vi "ex_readRawDataTDM.vi"(1 "read info in":T2, 5 "single values":bool, 7 "specified size":bool, 9 "segment size":i32, 11 "error in (no error)":errorcluster) -> (2 "read info out":T2, 6 "signals":waveform(dbl)[](array[waveform]), 10 "error out":errorcluster)   [LabVIEW 2017]
uses:
  <vilib>/Platform/express/TDMExpress.llb/ex_readInfoTDM.ctl
  <vilib>/Platform/express/TDMExpress.llb/ex_readChannelInfo.ctl
  <vilib>/express/express shared/ExFile.llb/ex_TdmData.ctl
  <vilib>/express/express shared/ExFile.llb/ex_TdmProperty.ctl
  <vilib>/express/express shared/ex_EditUserDefinedProperties/usiDataType.ctl
panel:
  out "x < y? 2":bool[](array[boolean])
  in  "Array 2":T1[](array[typedef])
  out "x*y":u32
  out "x < y?":bool[](array[boolean])
  out "data channel length":u32[](array[numeric])
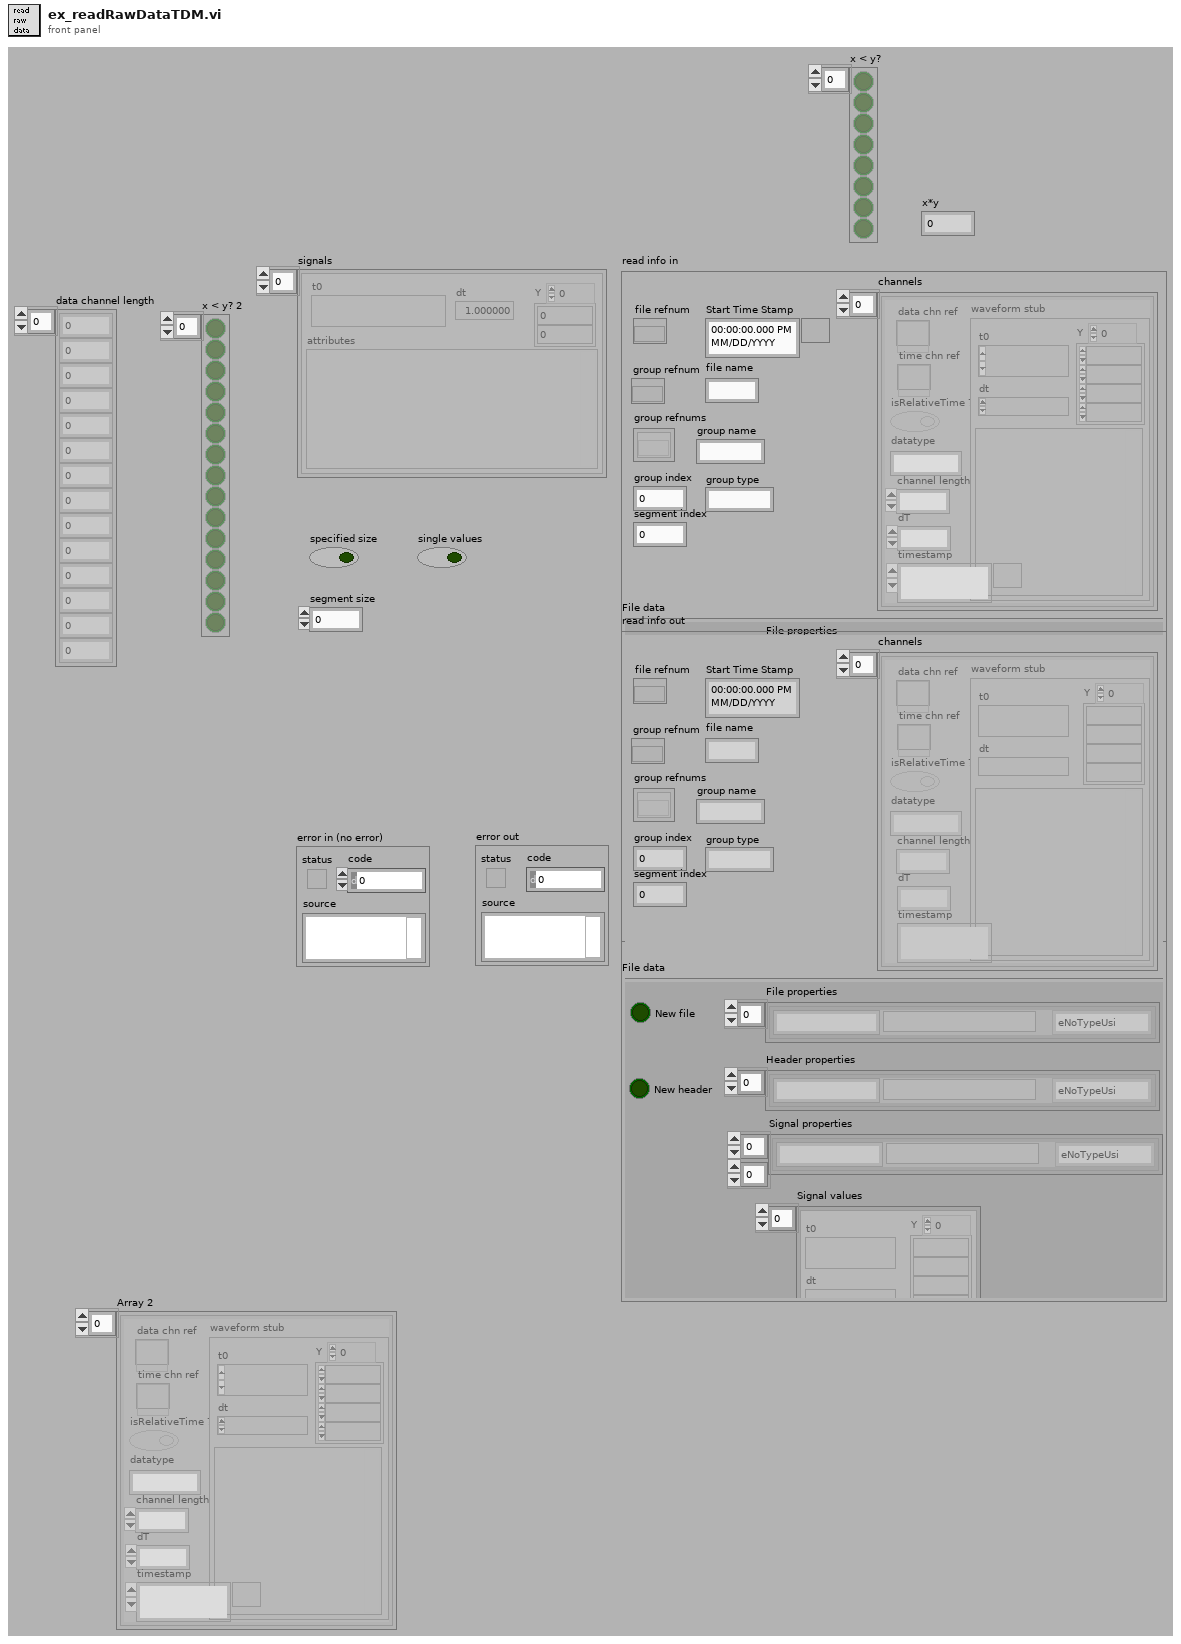
[diagram p1: front panel]
types:
  T1 = typedef "ex_readChannelInfo.ctl" = cluster{"data chn ref":refnum<k20>, "time chn ref":refnum<k20>, "isRelativeTime ?":bool, "channel length":u32, "dT":dbl, "waveform stub":waveform(dbl), "datatype":string, "timestamp":timestamp}
  T2 = typedef "ex_readInfoTDM.ctl" = cluster{"file refnum":refnum<k20>, "group refnum":refnum<k20>, "group name":string, "group type":string, "Start Time Stamp":timestamp, "group index":u32, "group refnums":refnum<k20>[], "file name":string, "segment index":u32, "channels":T1[], "File data":T3}
  T3 = typedef "ex_TdmData.ctl" = cluster{"New file":bool, "New header":bool, "File properties":T4[], "Header properties":T4[], "Signal properties":T4[][], "Signal values":waveform(dbl)[]}
  T4 = typedef "ex_TdmProperty.ctl" = cluster{"Name":string, "Type":T5, "Value":variant}
  T5 = typedef "usiDataType.ctl" = enum16{"eNoTypeUsi", "eInt8Usi", "eInt16Usi", "eInt32Usi", "eInt64Usi", "eUInt8Usi", "eUInt16Usi", "eUInt32Usi", "eUInt64Usi", "eFloat32Usi", "eFloat64Usi", "- 0", "- 1", "- 2", "- 3", "- 4", "- 5", "- 6", "- 7", "- 8", "- 9", "eString8Usi", "eString16Usi", "eStringUsi", "eEnumUsi", "- 10", "- 11", "- 12", "- 13", "- 14", "eTimeUsi", "- 15", "- 16", "- 17", "- 18", "- 19", "- 20", "- 21", "- 22", "- 23", "eInstanceUsi", "eStoreUsi"}
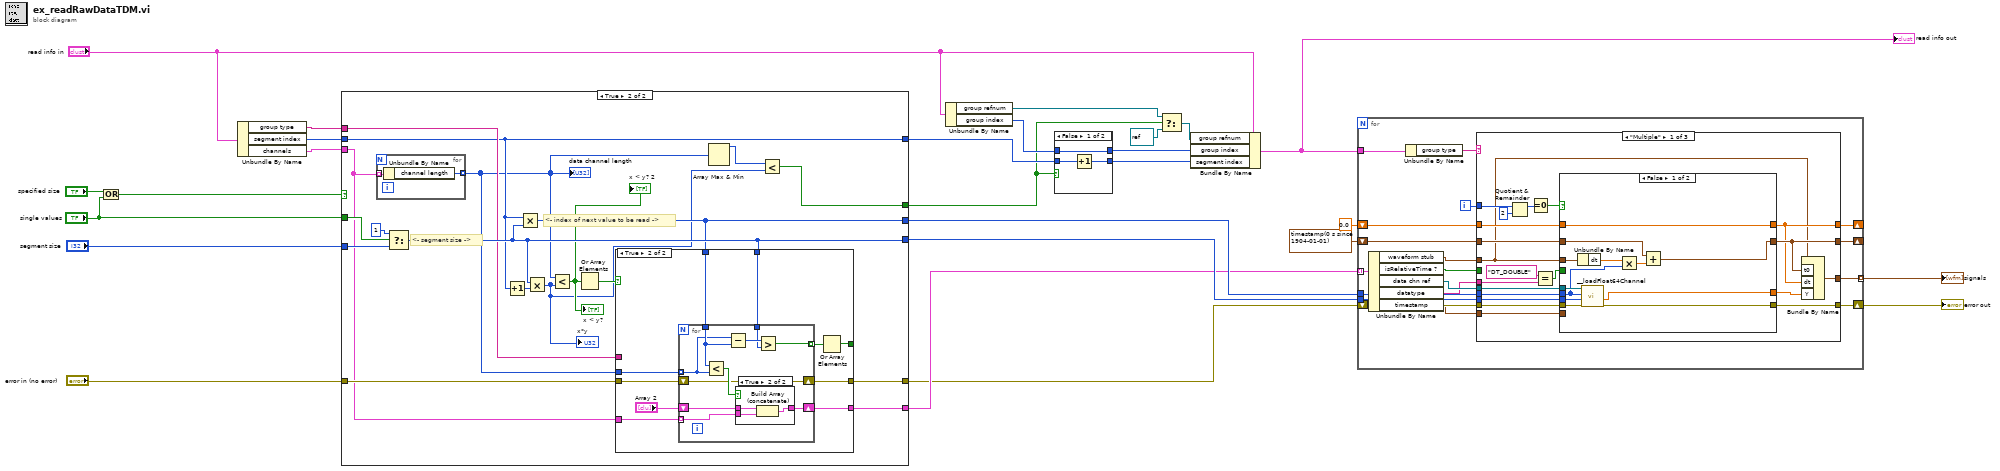
[diagram p0: block diagram]
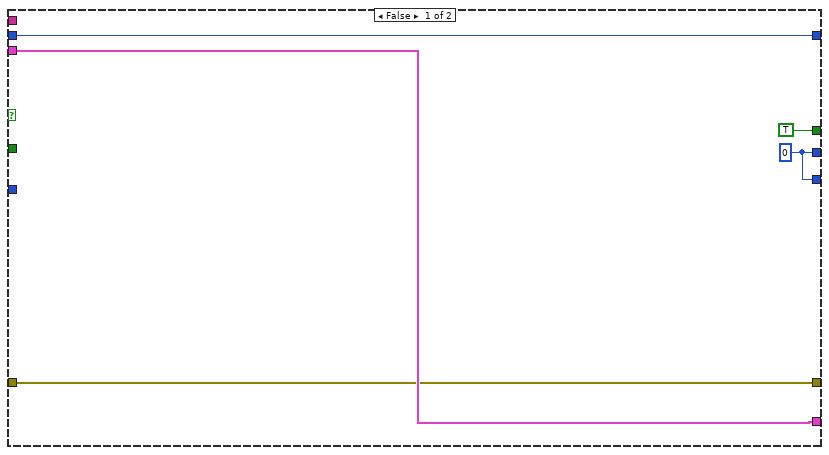
[diagram p2: hidden frame]
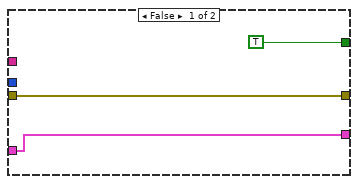
[diagram p3: hidden frame]
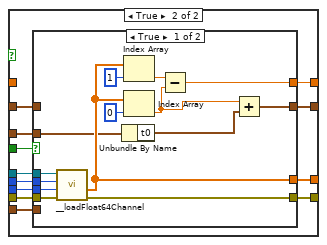
[diagram p5: hidden frame]
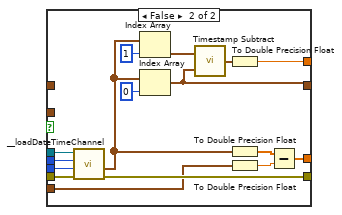
[diagram p6: hidden frame]
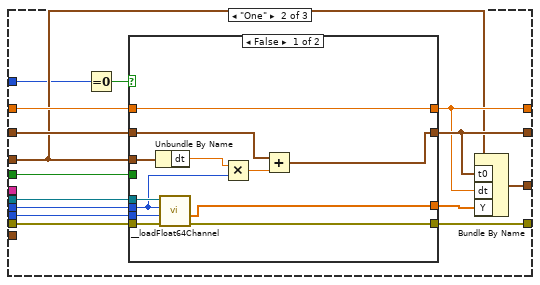
[diagram p7: hidden frame]
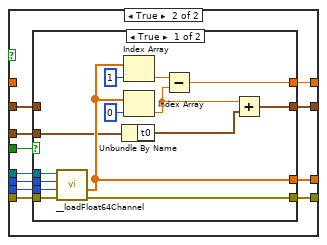
[diagram p8: hidden frame]
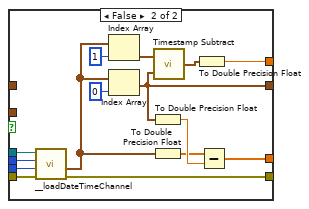
[diagram p9: hidden frame]
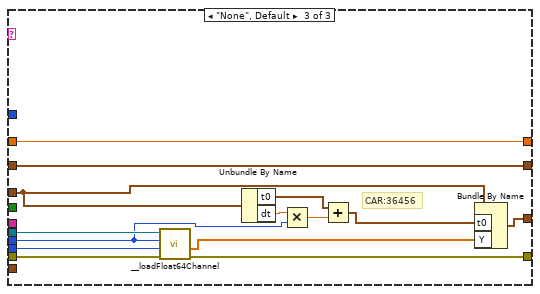
[diagram p10: hidden frame]
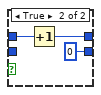
[diagram p11: hidden frame]
diagram:
  n1 = Or(x="specified size", y="single values") -> (x .or. y?=w20:bool)
  n2 = Unbundle By Name("read info in") -> ("group type"=w9:string, "segment index"=w6:u32, "channels"=w12:T1[])
  n3 = case shown="True" w20 {
    tunnel: "segment size" -> [_ w48]
    tunnel: "single values" -> [_ w47]
    tunnel: "error in (no error)" -> [w30 w46]
    tunnel: [w29 w44] -> w14
    tunnel: [TRUE w32] -> w1
    tunnel: [w29 w42] -> w13
    tunnel: [w30 w41] -> w2
    tunnel: w12 -> [w31 w39]
    tunnel: [w31 w38] -> w11
    tunnel: w9 -> [_ w37]
    tunnel: [w27 w36] -> w7
    tunnel: w6 -> [w27 w36]
    frame False {
      w29 = 0
    }
    frame True {
      # "<- index of next value to be read ->"
      # "<- segment size ->"
      n4 = for {
        tunnel: w39 -> [w51] mode=indexing
        tunnel: [w50] -> w35 mode=indexing
        n5 = Unbundle By Name(w51) -> ("channel length"=w50:u32)
      }
      "data channel length" <- w35
      n6 = Select(t=1, s=w47, f=w48) -> (s? t:f=w44:i32)
      n7 = Increment(x=w36) -> (x+1=w45:u32)
      n8 = Multiply(x=w36, y=w44) -> (x*y=w42:u32)
      n9 = Multiply(x=w44, y=w45) -> (x*y=w33:u32)
      "x*y" <- w33
      n10 = Less?(x=w35, y=w33) -> (x < y?=w43:bool[])
      "x < y?" <- w43
      "x < y? 2" <- w43
      n11 = Or Array Elements(Boolean array=w43) -> (logical OR=w40:bool)
      n12 = case shown="True" w40 {
        tunnel: w42 -> [_ w64]
        tunnel: [w54 w63] -> w41
        tunnel: [w53 w62] -> w38
        tunnel: [TRUE w57] -> _
        tunnel: w46 -> [w54 w61]
        tunnel: w37 -> [_ _]
        tunnel: w39 -> [w53 w60]
        tunnel: w44 -> [_ w59]
        tunnel: w35 -> [_ w55]
        frame False {
        }
        frame True {
          n13 = for {
            tunnel: w64 -> [w71]
            tunnel: w60 -> [w66] mode=indexing
            tunnel: w59 -> [w69]
            shift-right: [w73] -> w62
            shift-left: "Array 2" -> [w74]
            tunnel: [w68] -> w58 mode=indexing
            shift-right: [w67] -> w63
            shift-left: w61 -> [w67]
            tunnel: w55 -> [w65] mode=indexing
            n14 = Less?(x=w71, y=w65) -> (x < y?=w72:bool)
            n15 = Subtract(x=w65, y=w71) -> (x-y=w70:u32)
            n16 = case shown="True" w72 {
              tunnel: w74 -> [w75 w78]
              tunnel: w66 -> [_ w77]
              tunnel: [w75 w76] -> w73
              frame False {
              }
              frame True {
                n17 = Build Array (concatenate)(w78, w77) -> (w76:T1[])
              }
            }
            n18 = Greater?(x=w70, y=w69) -> (0:w68:bool)
          }
          n19 = Or Array Elements(Boolean array=w58) -> (logical OR=w57:bool)
        }
      }
      n20 = Array Max & Min(array=w35) -> (max value=w34:u32)  [unwired: 3 out]
      n21 = Less?(x=w34, y=w33) -> (x < y?=w32:bool)
    }
  }
  n22 = Unbundle By Name("read info in") -> ("group refnum"=w10:refnum<k20>, "group index"=w8:u32)
  n23 = case shown="False" w1 {
    tunnel: [w81 u32 0] -> w18
    tunnel: w7 -> [w80 _]
    tunnel: w8 -> [w79 w84]
    tunnel: [w79 w83] -> w17
    frame False {
      n24 = Increment(x=w80) -> (x+1=w81:u32)
    }
    frame True {
      n25 = Increment(x=w84) -> (x+1=w83:u32)
    }
  }
  n26 = Select(t=w10, s=w1, f=refnum<k20> refnum) -> (s? t:f=w15:refnum<k20>)
  n27 = Bundle By Name(cluster="read info in", "group refnum"=w15, "group index"=w17, "segment index"=w18) -> (w5:T2)
  "read info out" <- w5
  n28 = for {
    tunnel: w11 -> [w102] mode=indexing
    tunnel: w14 -> [w99]
    tunnel: w13 -> [w98]
    shift-right: [w87] -> w24
    shift-left: w2 -> [w100]
    tunnel: [w90] -> w25 mode=indexing
    shift-right: [w88] -> _
    shift-left: 0.0 -> [w92]
    tunnel: w5 -> [w101]
    shift-right: [w89] -> _
    shift-left: timestamp(0 s since 1904-01-01) -> [w93]
    i -> [w86]
    n29 = Unbundle By Name(w102) -> ("waveform stub"=w94:waveform(dbl), "isRelativeTime ?"=w96:bool, "data chn ref"=w97:refnum<k20>, "datatype"=w95:string, "timestamp"=w85:timestamp)
    n30 = Unbundle By Name(w101) -> ("group type"=w91:string)
    n31 = case shown="\"Multiple\"" w91 {
      tunnel: [w108 w179 w257] -> w88
      tunnel: w86 -> [w121 w177 _]
      tunnel: w92 -> [w118 w190 w257]
      tunnel: [w115 w187 w256] -> w89
      tunnel: w93 -> [w117 w189 w256]
      tunnel: w94 -> [w107 w178 w250]
      tunnel: [w116 w188 w255] -> w90
      tunnel: w100 -> [w111 w183 w253]
      tunnel: [w110 w182 w252] -> w87
      tunnel: w97 -> [w114 w186 w254]
      tunnel: w98 -> [w113 w185 w247]
      tunnel: w99 -> [w112 w184 w248]
      tunnel: w96 -> [_ w180 _]
      tunnel: w95 -> [w106 _ _]
      tunnel: w85 -> [w103 _ _]
      frame "Multiple" {
        n32 = Quotient & Remainder(x=w121, y=2) -> (x-y*floor(x/y)=w120:i32)  [unwired: 1 out]
        n33 = Equal To 0?(x=w120) -> (x = 0?=w119:bool)
        n34 = Equal?(x="DT_DOUBLE", y=w106) -> (x = y?=w105:bool)
        n35 = case shown="False" w119 {
          tunnel: [w129 w146] -> w108
          tunnel: w118 -> [w129 _]
          tunnel: [w123 w145] -> w115
          tunnel: w117 -> [w124 w138]
          tunnel: w114 -> [w134 w144]
          tunnel: w113 -> [w127 w143]
          tunnel: w112 -> [w133 w142]
          tunnel: w111 -> [w132 w141]
          tunnel: [w131 w140] -> w110
          tunnel: [w130 w139] -> w109
          tunnel: w105 -> [_ w136]
          tunnel: w107 -> [w128 w137]
          tunnel: w103 -> [_ w135]
          frame False {
            n36 = Unbundle By Name(w128) -> ("dt"=w126:dbl)
            n37 = call <vilib>:"__loadFloat64Channel.vi"("error in (no error)"=w132, "Count"=w133, "Index"=w127, "Data object in"=w134) -> ("error out"=w131:errorcluster, "Values"=w130:dbl[])  [unwired: 2 out]
            n38 = Multiply(x=w126, y=w127) -> (x*y=w125:dbl)
            n39 = Add(x=w124, y=w125) -> (x+y=w123:timestamp)
          }
          frame True {
            n40 = case shown="True" w136 {
              tunnel: [w152 w167] -> w146
              tunnel: [w148 w162] -> w145
              tunnel: w144 -> [w157 w174]
              tunnel: w143 -> [w151 w173]
              tunnel: w142 -> [w156 w172]
              tunnel: w141 -> [w155 w171]
              tunnel: [w154 w170] -> w140
              tunnel: [w153 w164] -> w139
              tunnel: w138 -> [_ _]
              tunnel: w137 -> [w150 _]
              tunnel: w135 -> [_ w161]
              frame True {
                n41 = call <vilib>:"__loadFloat64Channel.vi"("error in (no error)"=w155, "Count"=w156, "Index"=w151, "Data object in"=w157) -> ("error out"=w154:errorcluster, "Values"=w153:dbl[])  [unwired: 2 out]
                n42 = Unbundle By Name(w150) -> ("t0"=w149:timestamp)
                n43 = Index Array(array=w153, index=1) -> (element=w158:dbl)
                n44 = Index Array(array=w153, index=0) -> (element=w147:dbl)
                n45 = Subtract(x=w158, y=w147) -> (x-y=w152:dbl)
                n46 = Add(x=w147, y=w149) -> (x+y=w148:timestamp)
              }
              frame False {
                n47 = call <vilib>:"__loadDateTimeChannel.vi"("error in (no error)"=w171, "Count"=w172, "Index"=w173, "Data object in"=w174) -> ("error out"=w170:errorcluster, "Values"=w169:timestamp[])  [unwired: 2 out]
                n48 = Index Array(array=w169, index=1) -> (element=w168:timestamp)
                n49 = Index Array(array=w169, index=0) -> (element=w162:timestamp)
                n50 = call <vilib>:"Timestamp Subtract.vi"("y"=w162, "x"=w168) -> ("x - y"=w163:timestamp)
                n51 = To Double Precision Float(number=w163) -> (double precision float=w167:dbl)
                n52 = To Double Precision Float(number=w169) -> (double precision float=w165:dbl[])
                n53 = To Double Precision Float(number=w161) -> (double precision float=w166:dbl)
                n54 = Subtract(x=w165, y=w166) -> (x-y=w164:dbl[])
              }
            }
          }
        }
        n55 = Bundle By Name(cluster=w107, "t0"=w115, "dt"=w108, "Y"=w109) -> (w116:waveform(dbl))
      }
      frame "One" {
        n56 = Equal To 0?(x=w177) -> (x = 0?=w191:bool)
        n57 = case shown="False" w191 {
          tunnel: [w200 w214] -> w179
          tunnel: w190 -> [w200 _]
          tunnel: [w192 w213] -> w187
          tunnel: w189 -> [w193 w205]
          tunnel: w186 -> [w197 w212]
          tunnel: w185 -> [w196 w211]
          tunnel: w184 -> [w198 w210]
          tunnel: w183 -> [w203 w209]
          tunnel: [w202 w208] -> w182
          tunnel: [w201 w207] -> w181
          tunnel: w180 -> [_ w206]
          tunnel: w178 -> [w194 w204]
          frame False {
            n58 = Unbundle By Name(w194) -> ("dt"=w199:dbl)
            n59 = call <vilib>:"__loadFloat64Channel.vi"("error in (no error)"=w203, "Count"=w198, "Index"=w196, "Data object in"=w197) -> ("error out"=w202:errorcluster, "Values"=w201:dbl[])  [unwired: 2 out]
            n60 = Multiply(x=w199, y=w196) -> (x*y=w195:dbl)
            n61 = Add(x=w193, y=w195) -> (x+y=w192:timestamp)
          }
          frame True {
            n62 = case shown="True" w206 {
              tunnel: [w220 w233] -> w214
              tunnel: [w216 w232] -> w213
              tunnel: w212 -> [w225 w241]
              tunnel: w211 -> [w219 w240]
              tunnel: w210 -> [w224 w239]
              tunnel: w209 -> [w223 w238]
              tunnel: [w222 w237] -> w208
              tunnel: [w221 w229] -> w207
              tunnel: w205 -> [_ _]
              tunnel: w204 -> [w218 _]
              frame True {
                n63 = call <vilib>:"__loadFloat64Channel.vi"("error in (no error)"=w223, "Count"=w224, "Index"=w219, "Data object in"=w225) -> ("error out"=w222:errorcluster, "Values"=w221:dbl[])  [unwired: 2 out]
                n64 = Unbundle By Name(w218) -> ("t0"=w217:timestamp)
                n65 = Index Array(array=w221, index=1) -> (element=w226:dbl)
                n66 = Index Array(array=w221, index=0) -> (element=w215:dbl)
                n67 = Subtract(x=w226, y=w215) -> (x-y=w220:dbl)
                n68 = Add(x=w215, y=w217) -> (x+y=w216:timestamp)
              }
              frame False {
                n69 = call <vilib>:"__loadDateTimeChannel.vi"("error in (no error)"=w238, "Count"=w239, "Index"=w240, "Data object in"=w241) -> ("error out"=w237:errorcluster, "Values"=w236:timestamp[])  [unwired: 2 out]
                n70 = Index Array(array=w236, index=1) -> (element=w235:timestamp)
                n71 = Index Array(array=w236, index=0) -> (element=w232:timestamp)
                n72 = To Double Precision Float(number=w232) -> (double precision float=w231:dbl)
                n73 = To Double Precision Float(number=w236) -> (double precision float=w230:dbl[])
                n74 = call <vilib>:"Timestamp Subtract.vi"("y"=w232, "x"=w235) -> ("x - y"=w234:timestamp)
                n75 = To Double Precision Float(number=w234) -> (double precision float=w233:dbl)
                n76 = Subtract(x=w230, y=w231) -> (x-y=w229:dbl[])
              }
            }
          }
        }
        n77 = Bundle By Name(cluster=w178, "t0"=w187, "dt"=w179, "Y"=w181) -> (w188:waveform(dbl))
      }
      frame "None", Default {
        # "CAR:36456"
        n78 = call <vilib>:"__loadFloat64Channel.vi"("error in (no error)"=w253, "Count"=w248, "Index"=w247, "Data object in"=w254) -> ("error out"=w252:errorcluster, "Values"=w251:dbl[])  [unwired: 2 out]
        n79 = Unbundle By Name(w250) -> ("t0"=w245:timestamp, "dt"=w249:dbl)
        n80 = Multiply(x=w249, y=w247) -> (x*y=w246:dbl)
        n81 = Add(x=w245, y=w246) -> (x+y=w244:timestamp)
        n82 = Bundle By Name(cluster=w250, "t0"=w244, "Y"=w251) -> (w255:waveform(dbl))
      }
    }
  }
  "signals" <- w25
  "error out" <- w24
